vi "Decimation with IC.vi"(2 "initial decimation state":i32, 3 "init/cont (init:F)":bool, 4 "decimating factor (1)":i32=1 min=1 step=1, 5 "X":dbl[](array[numeric]) format="%.2f") -> (0 "final decimation state":i32, 1 "decimated X":dbl[](array[numeric]) format="%.2f")   [LabVIEW 2017]
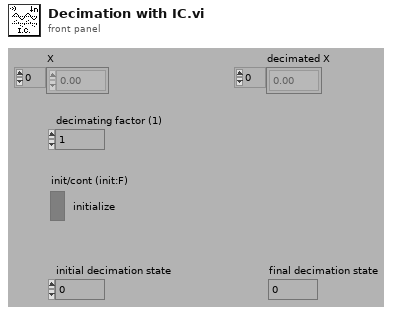
[diagram p1: front panel]
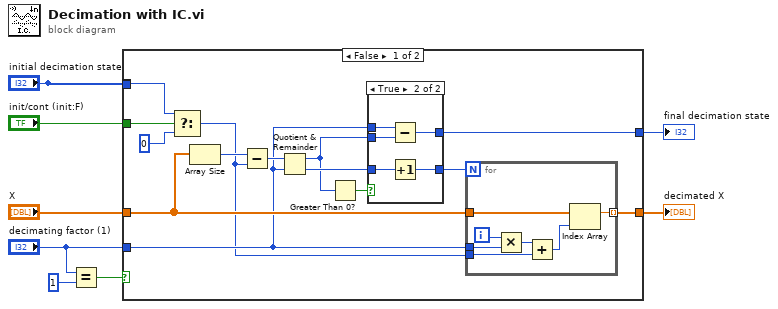
[diagram p0: block diagram]
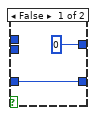
[diagram p2: hidden frame]
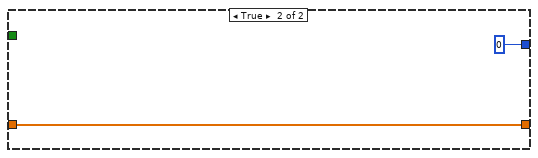
[diagram p3: hidden frame]
diagram:
  n1 = Equal?(x="decimating factor (1)", y=1) -> (x = y?=w4:bool)
  n2 = case shown="False" w4 {
    tunnel: [w9 w38] -> w8
    tunnel: "X" -> [w22 w38]
    tunnel: "initial decimation state" -> [_ _]
    tunnel: "decimating factor (1)" -> [w16 _]
    tunnel: [w14 0] -> w3
    tunnel: "init/cont (init:F)" -> [w12 _]
    tunnel: "initial decimation state" -> [w11 _]
    frame False {
      n3 = Select(t=w11, s=w12, f=0) -> (s? t:f=w13:i32)
      n4 = Array Size(array=w22) -> (size(s)=w20:i32)
      n5 = Subtract(x=w20, y=w13) -> (x-y=w21:i32)
      n6 = Quotient & Remainder(x=w21, y=w16) -> (x-y*floor(x/y)=w15:i32, floor(x/y)=w18:i32)
      n7 = Greater Than 0?(x=w15) -> (x > 0?=w19:bool)
      n8 = case shown="True" w19 {
        tunnel: w18 -> [w24 w29]
        tunnel: [w24 w28] -> w17
        tunnel: [0 w25] -> w14
        tunnel: w16 -> [_ w27]
        tunnel: w15 -> [_ w26]
        frame False {
        }
        frame True {
          n9 = Subtract(x=w27, y=w26) -> (x-y=w25:i32)
          n10 = Increment(x=w29) -> (x+1=w28:i32)
        }
      }
      n11 = for {
        N: w17 -> [_]
        tunnel: w16 -> [w35]
        tunnel: w22 -> [w36]
        tunnel: w13 -> [w31]
        tunnel: [w30] -> w9 mode=indexing
        i -> [w34]
        n12 = Multiply(x=w34, y=w35) -> (x*y=w33:i32)
        n13 = Add(x=w33, y=w31) -> (x+y=w32:i32)
        n14 = Index Array(array=w36, index=w32) -> (element=w30:dbl)
      }
    }
    frame True {
    }
  }
  "decimated X" <- w8
  "final decimation state" <- w3
